vi "Get ISO Time.vi"(8 "error in":errorcluster, 11 "LogRecord in":refnum<class "LogRecord.lvclass">) -> (0 "error out":errorcluster, 2 "ISO Time":string, 3 "LogRecord out":refnum<class "LogRecord.lvclass">)   [LabVIEW 2020, in "hse-logger.lvlib" / "LogRecord.lvclass"]
doc: "Returns the ISO-8601 formatted time of the LogRecord. \n\nDefault is with milliseconds.\n\n____\nHAMPEL SOFTWARE ENGINEERING v2.0.6 (2021-04-15 11:38)"
uses:
  LogRecord.lvclass
  LogRecord.lvclass/LogRecord.ctl
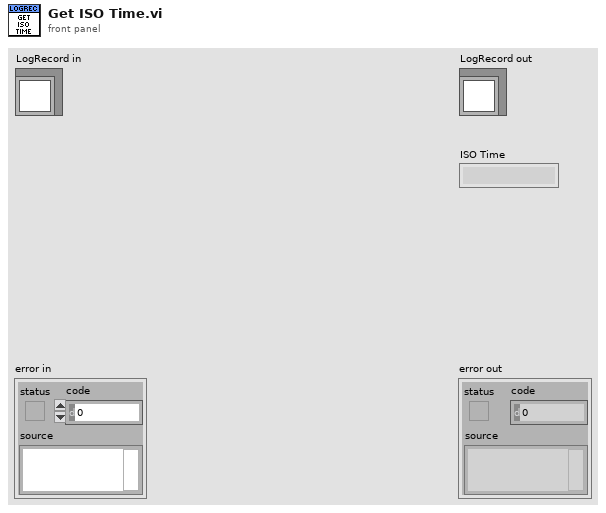
[diagram p1: front panel]
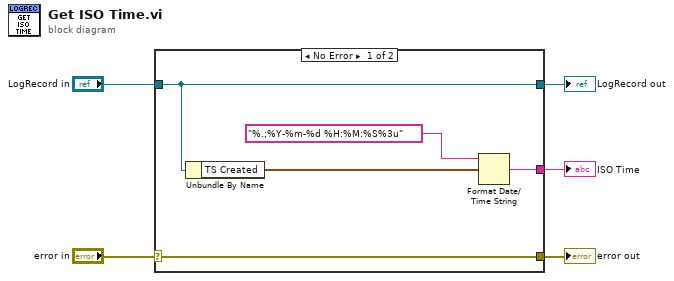
[diagram p0: block diagram]
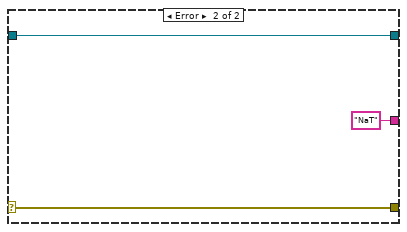
[diagram p2: hidden frame]
diagram:
  n1 = case shown="No Error" "error in" {
    selector: "error in" -> [w10 w12]
    tunnel: [w10 w12] -> w4
    tunnel: [w9 w13] -> w2
    tunnel: "LogRecord in" -> [w9 w13]
    tunnel: [w7 "NaT" ("date/time string")] -> w1
    frame No Error {
      n2 = Unbundle By Name(w9) -> ("TS Created"=w8:timestamp)
      n3 = Format Date/Time String(time format string (%c)="%.;%Y-%m-%d %H:%M:%S%3u", seconds (now)=w8) -> (date/time string=w7:string)  [unwired: 1 in]
    }
    frame Error {
    }
  }
  "error out" <- w4
  "LogRecord out" <- w2
  "ISO Time" <- w1
